vi "mboard eeprom get value.vi"(7 "strbuffer_len":u64, 8 "error in (no error)":errorcluster, 9 "value_out":string, 10 "key":string, 11 "h":u64) -> (0 "error out":errorcluster, 1 "value_out out":string, 3 "function return":u32(ring))   [LabVIEW 2023, in "uhd.lvlib"]
doc: "UHD_API uhd_error uhd_mboard_eeprom_get_value(\n uhd_mboard_eeprom_handle h, const char* key, char* value_out, size_t strbuffer_len);"
uses:
  <userlib>/uhd/uhd.lvlib
  <userlib>/uhd/uhd.dll
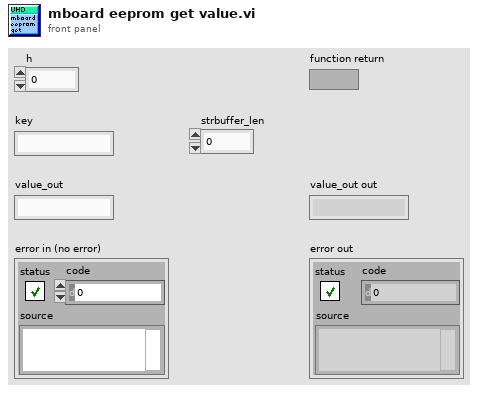
[diagram p1: front panel]
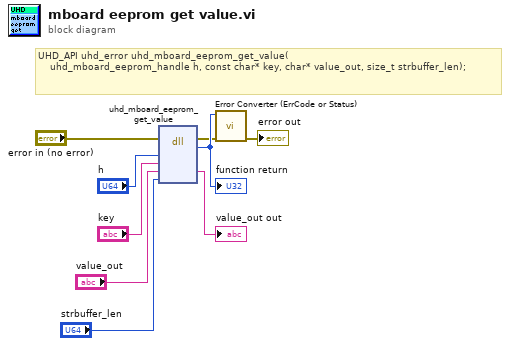
[diagram p0: block diagram]
diagram:
  # "UHD_API uhd_error uhd_mboard_eeprom_get_value(\n    uhd_mboard_eeprom_handle h, const char* key, char* value_out, size_t strbuffer_len);"
  n1 = dll-call lib="C:/Program Files/National Instruments/LabVIEW 2023/user.lib/uhd/uhd.*" fn="uhd_mboard_eeprom_get_value"(error in="error in (no error)", "h"="h", "key"="key", "value_out"="value_out", "strbuffer_len"="strbuffer_len") -> (error out=w2:errorcluster, w9:u32, "value_out"=→"value_out out":string)  [unwired: 5 in, 1 out]
  "function return" <- w9
  n2 = call <userlib>:"Error Converter (ErrCode or Status).vi"("error in (no error)"=w2, "error code"=w9) -> ("error out"=→"error out":errorcluster)  [unwired: 9 in]
